vi "Actor Core.vi"(8 "error in":errorcluster, 11 "Splitter Settings UI in":refnum<class "Splitter Settings UI.lvclass">) -> (0 "error out":errorcluster, 3 "Actor out":refnum<class "Actor.lvclass">)   [LabVIEW 2015, in "Splitter Settings UI.lvlib" / "Splitter Settings UI.lvclass"]
doc: "The user interface for this panel.\n\n----\nPlease see the following web address for additional documentation and tutorial information:\nhttp://www.mooregoodideas.com/mgi-panel-manager/\n\nAuthor: Derek Trepanier\n\nCopyright (c) 2018, Moore Good Ideas, Inc.\n\nAll rights reserved.\n\nRedistribution and use in source and binary forms, with or without modification, are permitted provided that the following conditions are met:\n\n * Redistributions of source code must retain the above copyright notice, this list of conditions and the following disclaimer.\n * Redistributions in binary form must reproduce the above copyright notice, this list of conditions and the following disclaimer in the documentation and/or other materials provided with the distribution.\n * Neither the name of Moore Good Ideas, Inc. nor the names of its contributors may be used to endorse or promote products derived from this software without specific prior written permission.\n\nTHIS SOFTWARE IS PROVIDED BY THE COPYRIGHT HOLDERS AND CONTRIBUTORS \"AS IS\" AND ANY EXPRESS OR IMPLIED WARRANTIES, INCLUDING, BUT NOT LIMITED TO, THE IMPLIED WARRANTIES OF MERCHANTABILITY AND FITNESS FOR A PARTICULAR PURPOSE ARE DISCLAIMED. IN NO EVENT SHALL THE COPYRIGHT OWNER OR CONTRIBUTORS BE LIABLE FOR ANY DIRECT, INDIRECT, INCIDENTAL, SPECIAL, EXEMPLARY, OR CONSEQUENTIAL DAMAGES (INCLUDING, BUT NOT LIMITED TO, PROCUREMENT OF SUBSTITUTE GOODS OR SERVICES; LOSS OF USE, DATA, OR PROFITS; OR BUSINESS INTERRUPTION) HOWEVER CAUSED AND ON ANY THEORY OF LIABILITY, WHETHER IN CONTRACT, STRICT LIABILITY, OR TORT (INCLUDING NEGLIGENCE OR OTHERWISE) ARISING IN ANY WAY OUT OF THE USE OF THIS SOFTWARE, EVEN IF ADVISED OF THE POSSIBILITY OF SUCH DAMAGE."
uses:
  Splitter Settings UI.lvclass
  <vilib>/ActorFramework/Actor/Actor.lvclass
  Typedefs/Splitter Style--Enum.ctl
  Splitter/Splitter.lvclass
  <vilib>/ActorFramework/Actor/Actor.lvclass/Actor.ctl
  <vilib>/ActorFramework/Message Enqueuer/Message Enqueuer.lvclass/Message Enqueuer.ctl
  Splitter Settings UI.lvclass/Splitter Settings UI.ctl
  Splitter Settings UI Messages/Set Cursor Busy State Msg/Set Cursor Busy State Msg.lvclass/Set Cursor Busy State Msg.ctl
  <vilib>/ActorFramework/Message Enqueuer/Init from Existing Queue.vi
  <vilib>/ActorFramework/Message Enqueuer/Enqueue.vi
  <vilib>/ActorFramework/Message Priority Queue/Priority Enqueue.vi
  <vilib>/ActorFramework/Message Enqueuer/Message Enqueuer.lvclass
  Pane Relief Main UI/Pane Relief Main UI Messages/Panel Object Settings Changed Msg/Panel Object Settings Changed Msg.lvclass
  Splitter Settings UI Messages/Set Cursor Busy State Msg/Set Cursor Busy State Msg.lvclass
  <vilib>/MGI/Panel Manager/Panel Actor/Panel Actor/Panel Actor.lvclass
panel:
  in  "Label":string
  in  "Style":T1 items=["Modern", "Classic", "System", "NXG"]
  in  "Size":i32 min=0
  in  "Color":u32(colorbox)
  in  "Locked":bool
  in  "Sticks":u16(ring) items=["Top", "Bottom", "Proportions"]
  in  "Position":i32
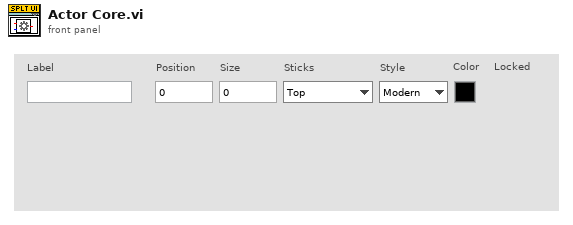
[diagram p1: front panel]
types:
  T1 = typedef "Splitter Style--Enum.ctl" = u16
  T2 = cluster{"Event Registration Refnum":refnum<event-registration>, "Pnl Actor":refnum<event-registration>}
  T3 = typedef "Splitter Sizing--Enum.ctl" = enum16{"Sticks Top/Left", "Sticks Bottom/Right", "Proportional"}
  T4 = typedef "Splitter Orientation--Enum.ctl" = enum16{"Vertical", "Horizontal"}
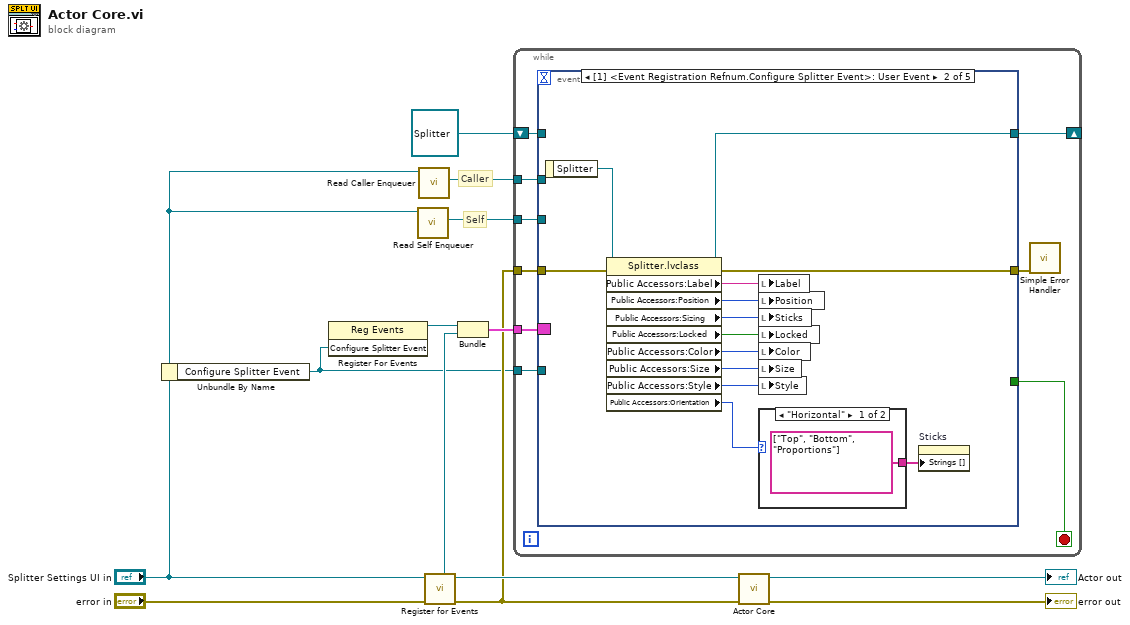
[diagram p0: block diagram]
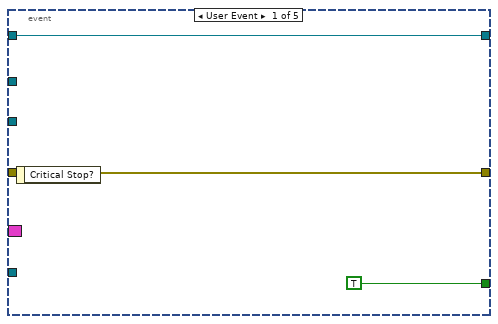
[diagram p2: hidden frame]
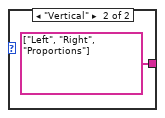
[diagram p3: hidden frame]
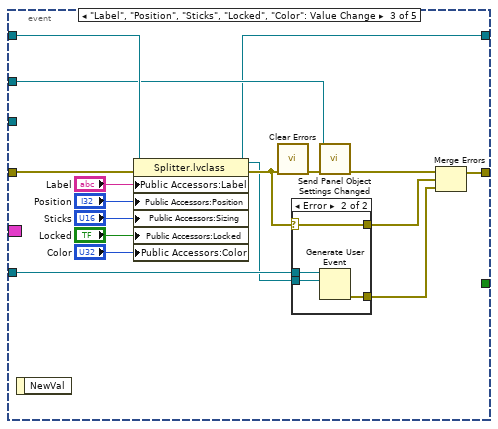
[diagram p4: hidden frame]
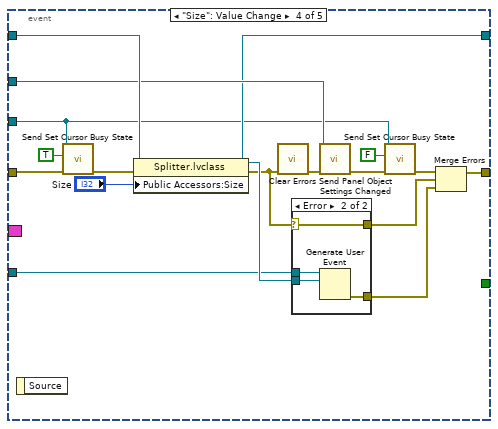
[diagram p6: hidden frame]
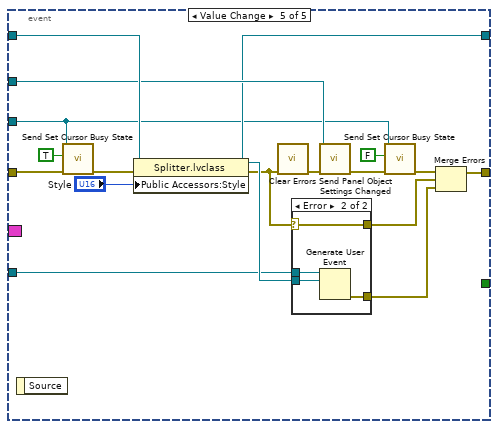
[diagram p8: hidden frame]
diagram:
  # "Self"
  # "Caller"
  n1 = Unbundle By Name("Splitter Settings UI in") -> ("Configure Splitter Event"=w3:refnum<user-event>)
  n2 = register-events(w3) -> (reference out=w9:refnum<event-registration>)  [unwired: 2 in, 1 out]
  n3 = call <vilib>:"Read Self Enqueuer.vi"("Actor"="Splitter Settings UI in") -> ("Self Enqueuer"=w2:refnum<class "Message Enqueuer.lvclass">)  [unwired: 10 in]
  n4 = call <vilib>:"Read Caller Enqueuer.vi"("Actor"="Splitter Settings UI in") -> ("Caller Enqueuer"=w4:refnum<class "Message Enqueuer.lvclass">)  [unwired: 10 in]
  n5 = call <vilib>:"Register for Events.vi"("Error In"="error in", "Panel Actor in"="Splitter Settings UI in") -> ("Error Out"=w5:errorcluster, "Panel Actor out"=w11:refnum<class "Splitter Settings UI.lvclass">, "Pnl Actor"=w8:refnum<event-registration>)  [unwired: 6 in, 1 out]
  n6 = Bundle("Event Registration Refnum"=w9, "Pnl Actor"=w8) -> (w7:T2)  [unwired: 1 in]
  n7 = while {
    tunnel: w7 -> [w22]
    shift-right: [w20] -> _
    shift-left: refnum<class "Splitter.lvclass"> refnum ("Splitter.lvclass") -> [w19]
    tunnel: w4 -> [w17]
    tunnel: w5 -> [w18]
    tunnel: w3 -> [w15]
    tunnel: w2 -> [w14]
    stop <- w21 stop-if-true
    n8 = event shown="[1] <Event Registration Refnum.Configure Splitter Event>: User Event" {
      selector: w22 -> [_ _ _ _ _]
      dyn-events: _ -> [_ _ _ _ _]
      timeout: _ -> [_ _ _ _ _]
      tunnel: [TRUE _ _ _ _] -> w21
      tunnel: [w25 w31 w42 w71 w94] -> w20
      tunnel: w19 -> [w25 _ w50 w78 w100]
      tunnel: w18 -> [w24 w33 w51 w66 w89]
      tunnel: [w24 w32 w46 w75 w98] -> w16
      tunnel: w17 -> [_ _ w48 w74 w97]
      tunnel: w15 -> [_ _ w43 w69 w92]
      tunnel: w14 -> [_ _ _ w64 w87]
      event User Event {
        n9 = event-data() -> ()  [unwired: 1 in, 1 out]
      }
      event User Event {
        n10 = event-data() -> ("Splitter"=w30:refnum<class "Splitter.lvclass">)  [unwired: 1 in]
        n11 = property class="Splitter.lvclass"(reference=w30, error in=w33) -> (reference out=w31:refnum<class "Splitter.lvclass">, error out=w32:errorcluster, "Public Accessors:Label"=w38:string, "Public Accessors:Position"=w37:i32, "Public Accessors:Sizing"=w36:T3, "Public Accessors:Locked"=w35:bool, "Public Accessors:Color"=w34:u32, "Public Accessors:Size"=w29:i32, "Public Accessors:Style"=w26:T1, "Public Accessors:Orientation"=w27:T4)
        n12 = local write "Label"(w38) -> ()
        n13 = local write "Position"(w37) -> ()
        n14 = local write "Sticks"(w36) -> ()
        n15 = local write "Locked"(w35) -> ()
        n16 = local write "Color"(w34) -> ()
        n17 = local write "Size"(w29) -> ()
        n18 = local write "Style"(w26) -> ()
        n19 = case shown="\"Horizontal\"" w27 {
          tunnel: [string[] ["Top", "Bottom", "Proportions"] ("Strings []") string[] ["Left", "Right", "Proportions"] ("Strings []")] -> w28
          frame "Horizontal" {
          }
          frame "Vertical" {
          }
        }
        n20 = property on="Sticks" class="Ring (strict)"("Strings []"=w28) -> ()  [unwired: 2 in, 2 out]
      }
      event "Label", "Position", "Sticks", "Locked", "Color": Value Change {
        n21 = event-data() -> ()  [unwired: 1 in, 1 out]
        n22 = property class="Splitter.lvclass"(reference=w50, error in=w51, "Public Accessors:Label"="Label", "Public Accessors:Position"="Position", "Public Accessors:Sizing"="Sticks", "Public Accessors:Locked"="Locked", "Public Accessors:Color"="Color") -> (reference out=w42:refnum<class "Splitter.lvclass">, error out=w44:errorcluster)
        n23 = call <vilib>:"Clear Errors.vi"("error in (no error)"=w44) -> ("error out"=w49:errorcluster)  [unwired: 5 in, 1 out]
        n24 = case shown="Error" w44 {
          selector: w44 -> [w57 w61]
          tunnel: [w57 w61] -> w45
          tunnel: w43 -> [_ w60]
          tunnel: w42 -> [_ w59]
          tunnel: [_ w58] -> w41
          frame No Error {
          }
          frame Error {
            n25 = Generate User Event(user event=w60, event data cluster=w59) -> (error out=w58:errorcluster)  [unwired: 2 in, 1 out]
          }
        }
        n26 = call "Send Panel Object Settings Changed.vi"("error in (no error)"=w49, "Message Enqueuer"=w48) -> ("error out"=w47:errorcluster)  [unwired: 8 in, 1 out]
        n27 = Merge Errors(w47, w45, w41) -> (w46:errorcluster)
      }
      event "Size": Value Change {
        n28 = event-data() -> ()  [unwired: 1 in, 1 out]
        n29 = call "Send Set Cursor Busy State.vi"("error in (no error)"=w66, "Busy?"=TRUE, "Message Enqueuer"=w64) -> ("error out"=w67:errorcluster)  [unwired: 7 in, 1 out]
        n30 = property class="Splitter.lvclass"(reference=w78, error in=w67, "Public Accessors:Size"="Size") -> (reference out=w71:refnum<class "Splitter.lvclass">, error out=w70:errorcluster)
        n31 = call <vilib>:"Clear Errors.vi"("error in (no error)"=w70) -> ("error out"=w76:errorcluster)  [unwired: 5 in, 1 out]
        n32 = case shown="Error" w70 {
          selector: w70 -> [w79 w83]
          tunnel: [w79 w83] -> w73
          tunnel: w69 -> [_ w82]
          tunnel: w71 -> [_ w81]
          tunnel: [_ w80] -> w72
          frame No Error {
          }
          frame Error {
            n33 = Generate User Event(user event=w82, event data cluster=w81) -> (error out=w80:errorcluster)  [unwired: 2 in, 1 out]
          }
        }
        n34 = call "Send Panel Object Settings Changed.vi"("error in (no error)"=w76, "Message Enqueuer"=w74) -> ("error out"=w63:errorcluster)  [unwired: 8 in, 1 out]
        n35 = call "Send Set Cursor Busy State.vi"("error in (no error)"=w63, "Busy?"=FALSE, "Message Enqueuer"=w64) -> ("error out"=w62:errorcluster)  [unwired: 7 in, 1 out]
        n36 = Merge Errors(w62, w73, w72) -> (w75:errorcluster)
      }
      event Value Change {
        n37 = event-data() -> ()  [unwired: 1 in, 1 out]
        n38 = call "Send Set Cursor Busy State.vi"("error in (no error)"=w89, "Busy?"=TRUE, "Message Enqueuer"=w87) -> ("error out"=w90:errorcluster)  [unwired: 7 in, 1 out]
        n39 = property class="Splitter.lvclass"(reference=w100, error in=w90, "Public Accessors:Style"="Style") -> (reference out=w94:refnum<class "Splitter.lvclass">, error out=w93:errorcluster)
        n40 = call <vilib>:"Clear Errors.vi"("error in (no error)"=w93) -> ("error out"=w99:errorcluster)  [unwired: 5 in, 1 out]
        n41 = case shown="Error" w93 {
          selector: w93 -> [w101 w105]
          tunnel: [w101 w105] -> w96
          tunnel: w92 -> [_ w104]
          tunnel: w94 -> [_ w103]
          tunnel: [_ w102] -> w95
          frame No Error {
          }
          frame Error {
            n42 = Generate User Event(user event=w104, event data cluster=w103) -> (error out=w102:errorcluster)  [unwired: 2 in, 1 out]
          }
        }
        n43 = call "Send Panel Object Settings Changed.vi"("error in (no error)"=w99, "Message Enqueuer"=w97) -> ("error out"=w86:errorcluster)  [unwired: 8 in, 1 out]
        n44 = call "Send Set Cursor Busy State.vi"("error in (no error)"=w86, "Busy?"=FALSE, "Message Enqueuer"=w87) -> ("error out"=w85:errorcluster)  [unwired: 7 in, 1 out]
        n45 = Merge Errors(w85, w96, w95) -> (w98:errorcluster)
      }
    }
    n46 = call <vilib>:"Simple Error Handler.vi"("error in (no error)"=w16) -> ()  [unwired: 4 in, 5 out]
  }
  n47 = call-parent "Actor Core.vi"("error in"=w5, "Panel Actor in"=w11) -> ("error out"=→"error out":errorcluster, "Actor out"=→"Actor out":refnum<class "Actor.lvclass">)  [unwired: 8 in]
